vi "Dummy TVC.vi"() -> ()   [LabVIEW 2025]
uses:
  controls/TED4015 Status.ctl
  <vilib>/addons/_JKI Toolkits/State Machine/_JKI_lib_State_Machine.llb/Select State(s)_err__jki_lib_state_machine.vi
  <vilib>/addons/_JKI Toolkits/State Machine/_JKI_lib_State_Machine.llb/Periodic Trigger__ogtk__JKI-SM__jki_lib_state_machine.vi
panel:
  in  "LED_Stimulate":bool
  in  "LED_Illuminate":bool
  in  "Heater Enable":bool
  in  "PSU Enable":bool
  in  "TLUP_Temperatures":waveform(dbl)[](array[waveform])=[{"t0"=timestamp(3820413812.102944 s since 1904-01-01), "dt"=1.0, "Y"=[23.56152], "attributes"=variant("NI_ChannelName"=variant(string "TLUP_0"))}, {"t0"=timestamp(3820413812.102944 s since 1904-01-01), "dt"=1.0, "Y"=[-999.0], "attributes"=variant("NI_ChannelName"=variant(string "TLUP_1"))}, {"t0"=timestamp(3820413812.102944 s since 1904-01-01), "dt"=1.0, "Y"=[-999.0], "attributes"=variant("NI_ChannelName"=variant(string "TLUP_2"))}, {"t0"=timestamp(3820413812.102944 s since 1904-01-01), "dt"=1.0, "Y"=[-999.0], "attributes"=variant("NI_ChannelName"=variant(string "TLUP_3"))}, {"t0"=timestamp(3820413812.102944 s since 1904-01-01), "dt"=1.0, "Y"=[nan], "attributes"=variant("NI_ChannelName"=variant(string "TLUP_4"))}, {"t0"=timestamp(3820413812.102944 s since 1904-01-01), "dt"=1.0, "Y"=[nan], "attributes"=variant("NI_ChannelName"=variant(string "TLUP_5"))}, {"t0"=timestamp(3820413812.102944 s since 1904-01-01), "dt"=1.0, "Y"=[nan], "attributes"=variant("NI_ChannelName"=variant(string "TLUP_6"))}, {"t0"=timestamp(3820413812.102944 s since 1904-01-01), "dt"=1.0, "Y"=[nan], "attributes"=variant("NI_ChannelName"=variant(string "TLUP_7"))}]
  in  "TEC On":bool[](array[boolean])=[FALSE, FALSE]
  in  "DS enabled?":bool
  in  "Exit":bool
  out "TVC_StopAfterCycle":bool
  out "TVC_CyclesRemaining":i32
  in  "TVC_CycleNumber":i32
  in  "Diode Currents":waveform(dbl)[](array[waveform])
  in  "TED Status":T1[](array[typedef])
  in  "PSU_Monitor":waveform(dbl)[](array[waveform])=[{"t0"=timestamp(3820413812.1099424 s since 1904-01-01), "dt"=1.0, "Y"=[2.52], "attributes"=variant("NI_ChannelName"=variant(string "Board_Voltage_0"))}, {"t0"=timestamp(3820413812.1153584 s since 1904-01-01), "dt"=1.0, "Y"=[-0.009], "attributes"=variant("NI_ChannelName"=variant(string "Board_Voltage_0"))}, {"t0"=timestamp(3820413812.1099424 s since 1904-01-01), "dt"=1.0, "Y"=[-0.017], "attributes"=variant("NI_ChannelName"=variant(string "Board_Current_0"))}, {"t0"=timestamp(3820413812.1153584 s since 1904-01-01), "dt"=1.0, "Y"=[0.0], "attributes"=variant("NI_ChannelName"=variant(string "Board_Current_0"))}]
  in  "Heater Monitor":waveform(dbl)[](array[waveform])=[{"t0"=timestamp(3820413812.092942 s since 1904-01-01), "dt"=1.0, "Y"=[-0.005], "attributes"=variant("NI_ChannelName"=variant(string "Heater_Voltage"))}, {"t0"=timestamp(3820413812.092942 s since 1904-01-01), "dt"=1.0, "Y"=[-0.002], "attributes"=variant("NI_ChannelName"=variant(string "Heater_Current"))}]
  in  "TVC_Temperatures":waveform(dbl)[](array[waveform])=[{"t0"=timestamp(3820413812.1049423 s since 1904-01-01), "dt"=1.0, "Y"=[-80.0], "attributes"=variant("NI_ChannelName"=variant(string "3A"))}, {"t0"=timestamp(3820413812.1049423 s since 1904-01-01), "dt"=1.0, "Y"=[0.1969585335155295], "attributes"=variant("NI_ChannelName"=variant(string "3B"))}, {"t0"=timestamp(3820413812.1049423 s since 1904-01-01), "dt"=1.0, "Y"=[0.2898606356704896], "attributes"=variant("NI_ChannelName"=variant(string "3C"))}, {"t0"=timestamp(3820413812.1049423 s since 1904-01-01), "dt"=1.0, "Y"=[0.3274623555028864], "attributes"=variant("NI_ChannelName"=variant(string "3D"))}, {"t0"=timestamp(3820413812.1049423 s since 1904-01-01), "dt"=1.0, "Y"=[0.3794250746071903], "attributes"=variant("NI_ChannelName"=variant(string "4A"))}, {"t0"=timestamp(3820413812.1049423 s since 1904-01-01), "dt"=1.0, "Y"=[0.7650917242886434], "attributes"=variant("NI_ChannelName"=variant(string "4B"))}, {"t0"=timestamp(3820413812.1049423 s since 1904-01-01), "dt"=1.0, "Y"=[0.4416685188806395], "attributes"=variant("NI_ChannelName"=variant(string "4C"))}, {"t0"=timestamp(3820413812.1049423 s since 1904-01-01), "dt"=1.0, "Y"=[0.7497510727682433], "attributes"=variant("NI_ChannelName"=variant(string "4D"))}, {"t0"=timestamp(3820413812.1049423 s since 1904-01-01), "dt"=1.0, "Y"=[0.8015992709050663], "attributes"=variant("NI_ChannelName"=variant(string "Target"))}]
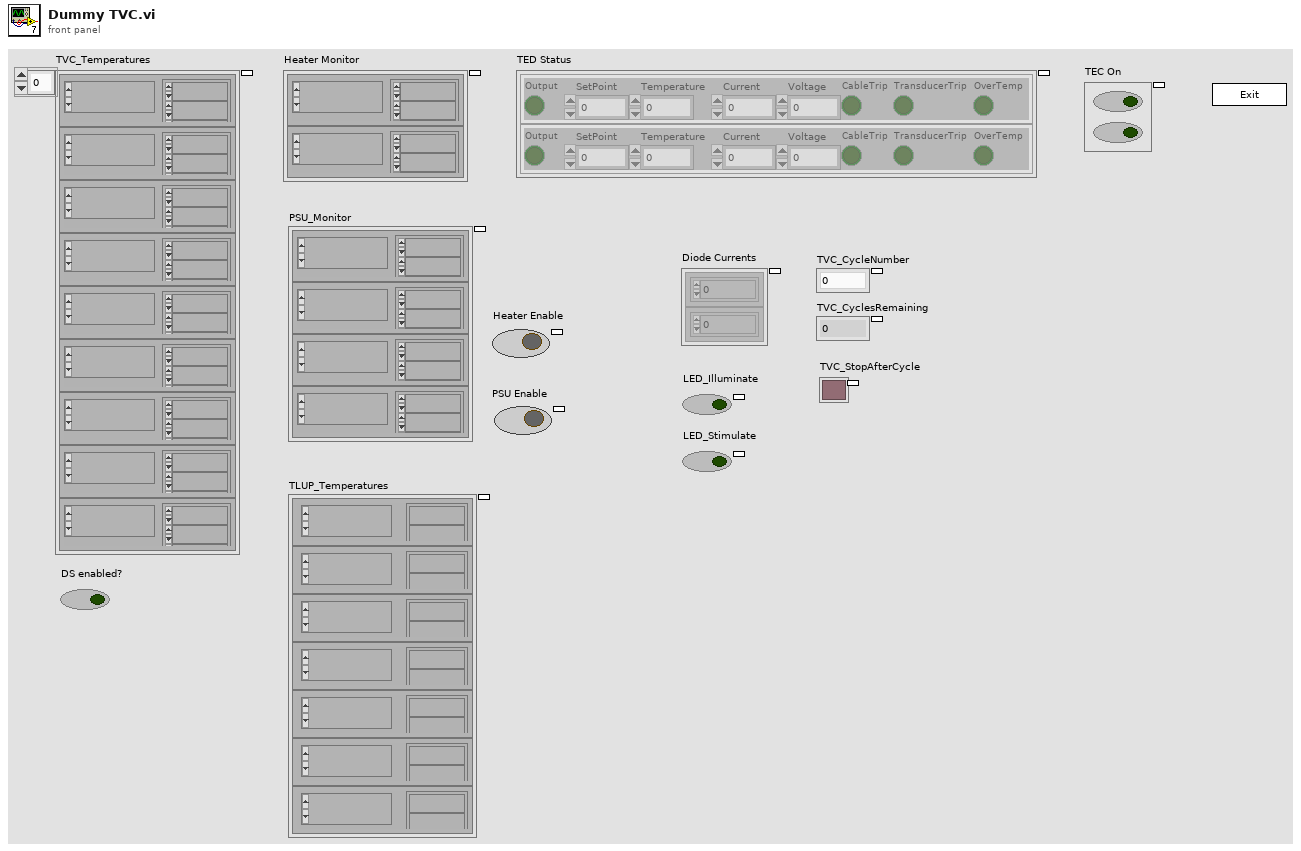
[diagram p1: front panel]
types:
  T1 = typedef "TED4015 Status.ctl" = cluster{"Output":bool, "SetPoint":dbl, "Temperature":dbl, "Current":dbl, "Voltage":dbl, "CableTrip":bool, "TransducerTrip":bool, "OverTemp":bool}
  T2 = enum32{"Invalid", "Standard", "Closed", "Hidden", "Minimized", "Maximized"}
  T3 = enum32{"invalid app kind", "Development System", "Run Time System", "Student Edition", "Embedded LabVIEW", "Evaluation", "Custom"}
  T4 = cluster{"Core":cluster{"Current VI Reference":refnum<vi>, "Close Panel on Exit?":bool}, "Your Boolean data":bool, "Your string data":string}
  T5 = cluster{"Current VI Reference":refnum<vi>, "Close Panel on Exit?":bool}
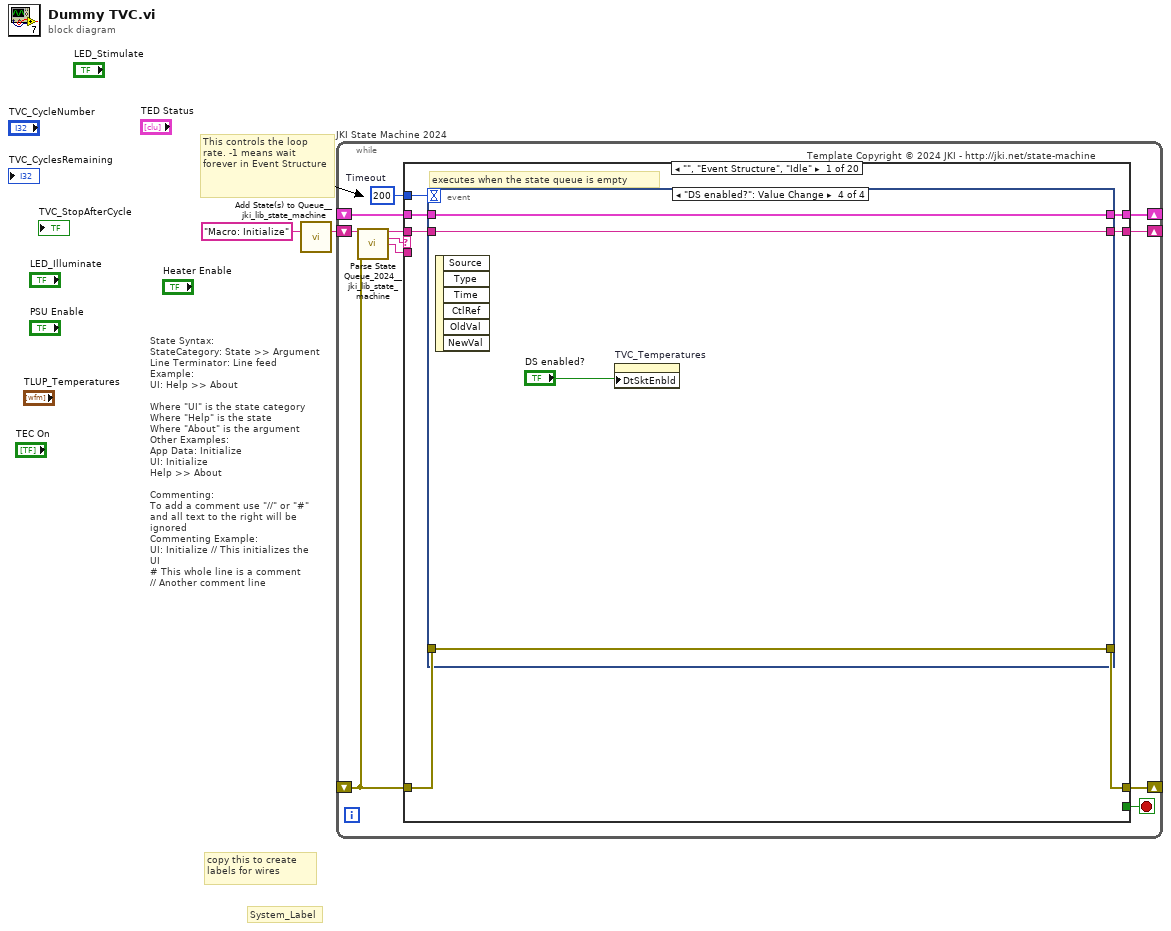
[diagram p0: block diagram]
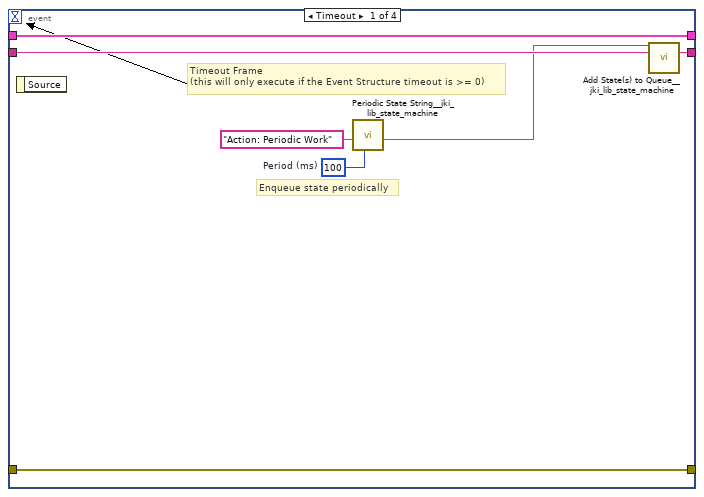
[diagram p2: hidden frame]
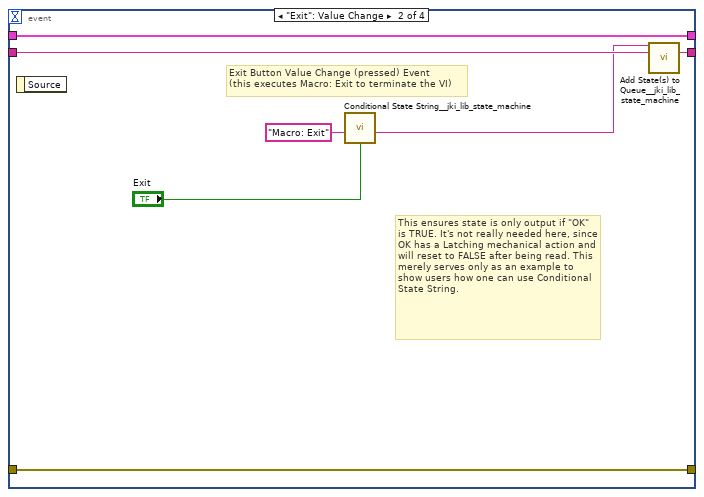
[diagram p3: hidden frame]
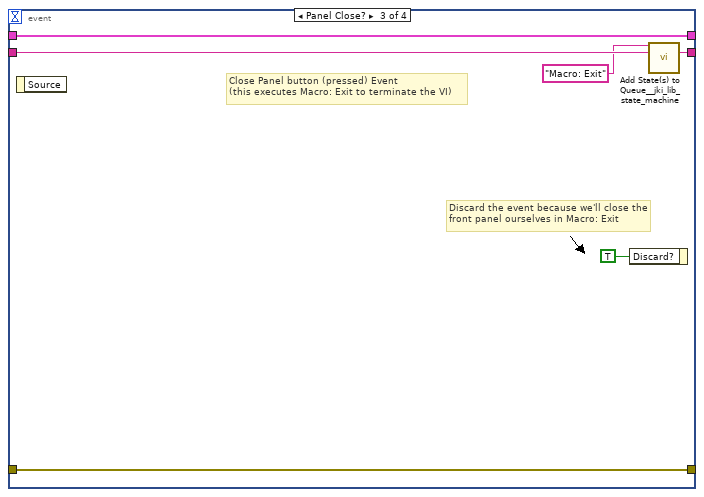
[diagram p4: hidden frame]
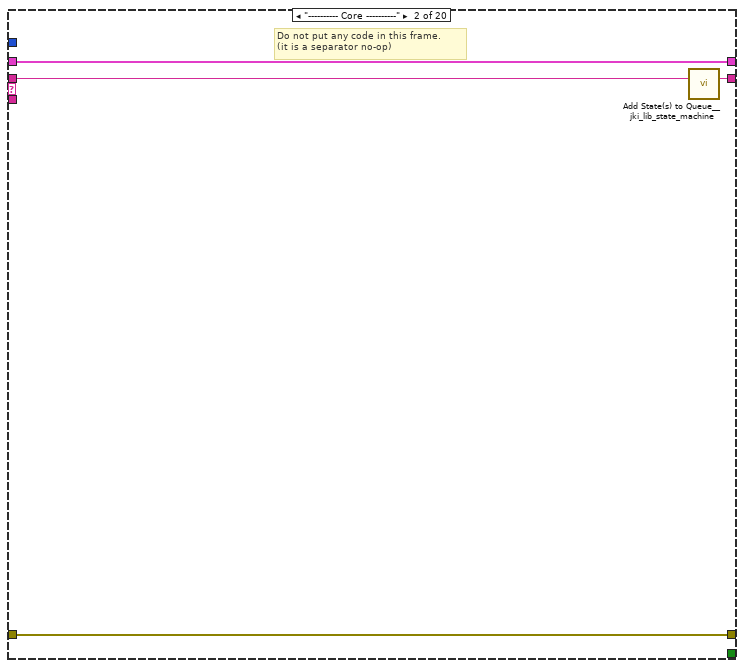
[diagram p5: hidden frame]
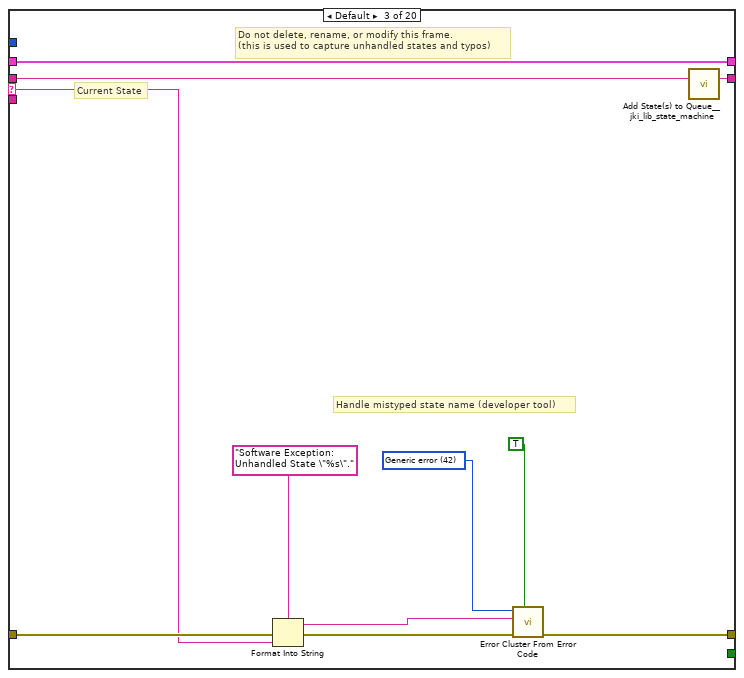
[diagram p6: hidden frame]
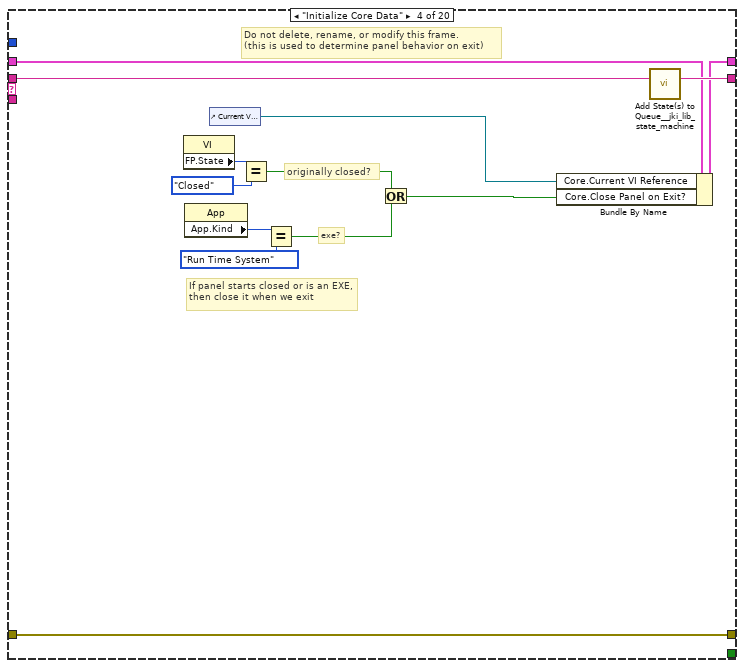
[diagram p7: hidden frame]
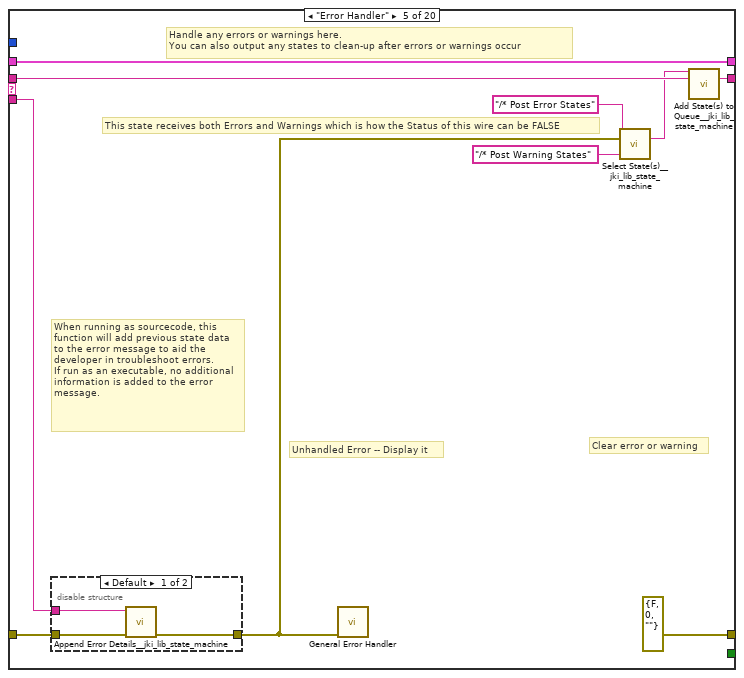
[diagram p8: hidden frame]
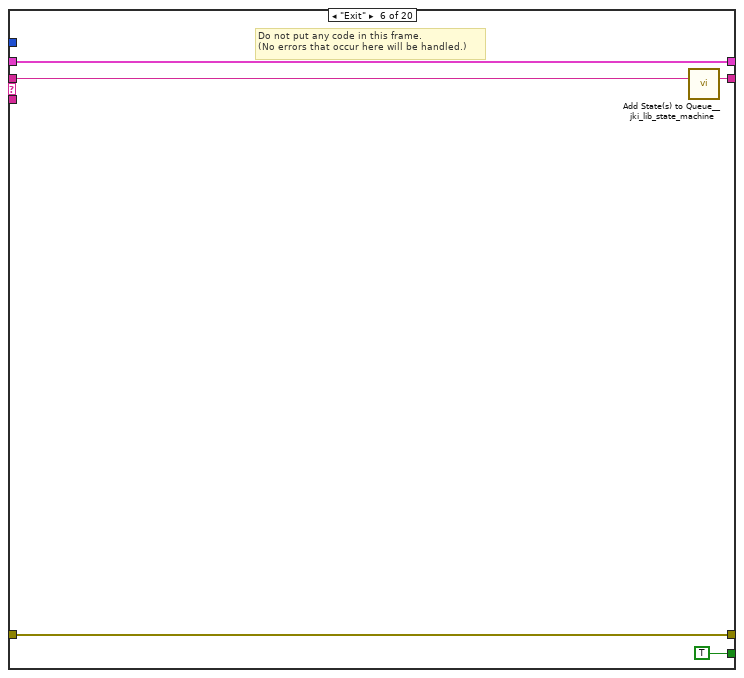
[diagram p10: hidden frame]
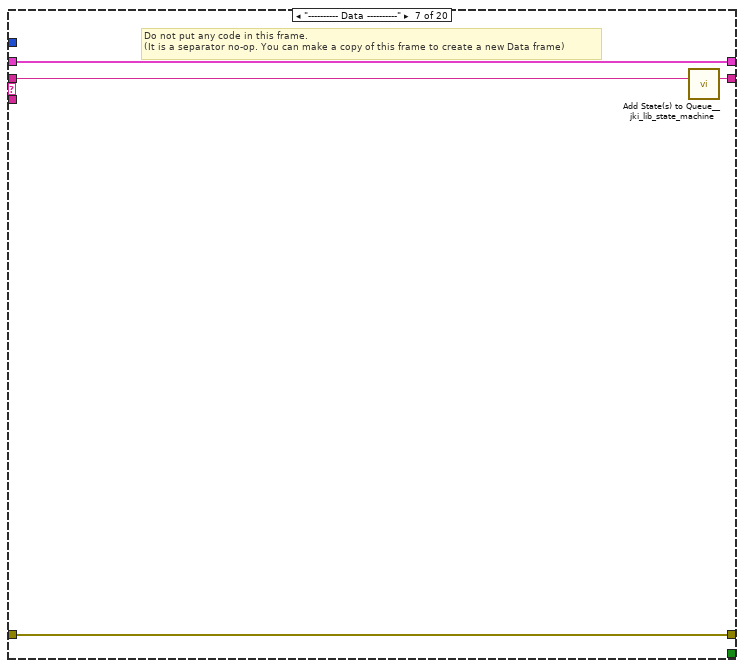
[diagram p11: hidden frame]
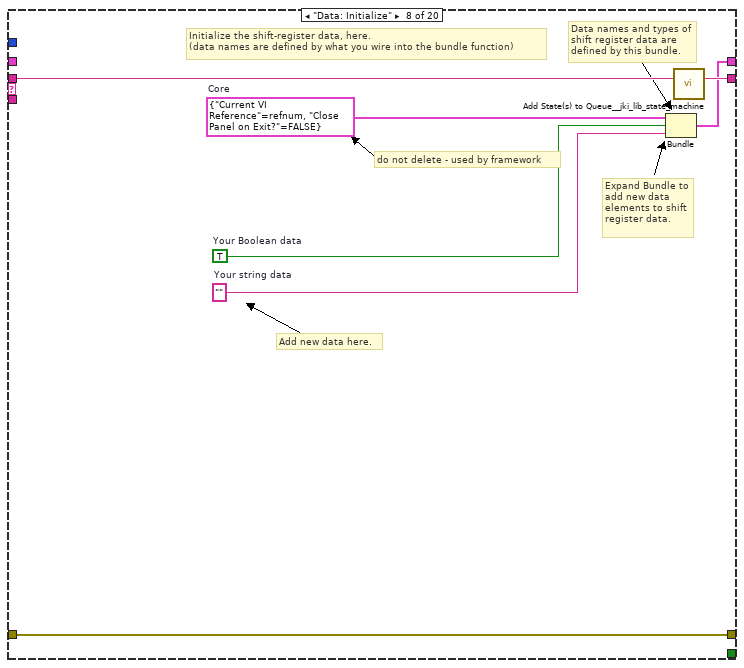
[diagram p12: hidden frame]
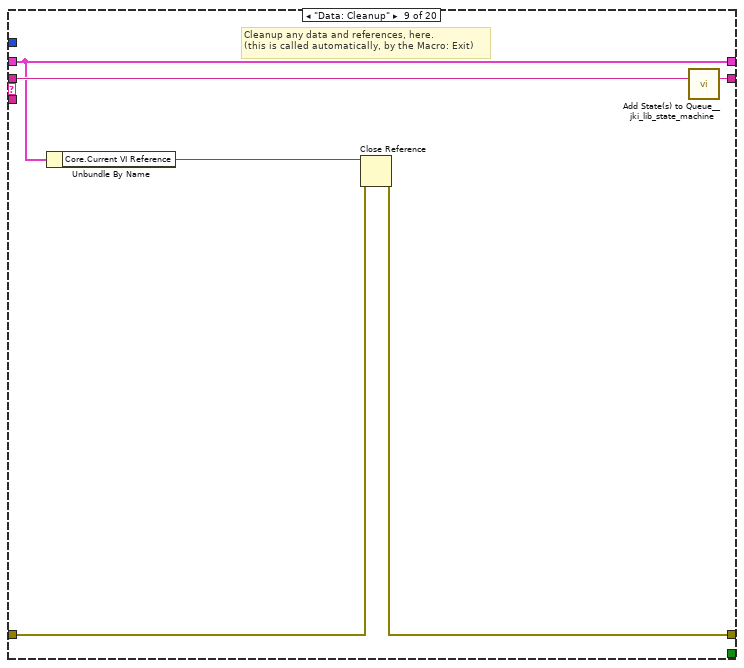
[diagram p13: hidden frame]
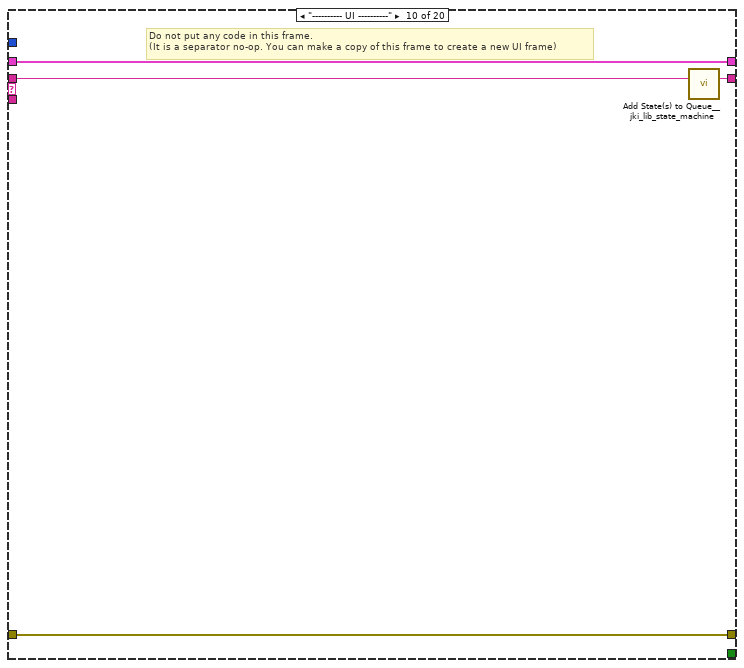
[diagram p14: hidden frame]
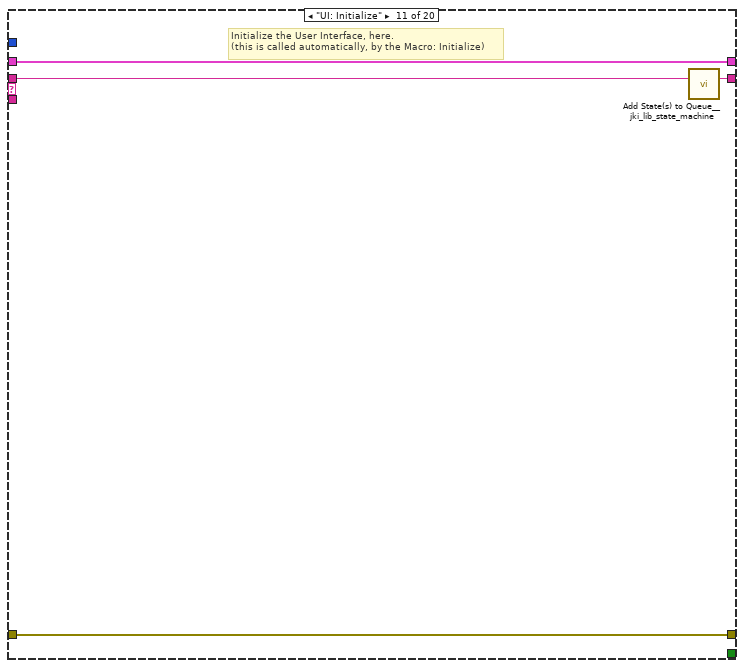
[diagram p15: hidden frame]
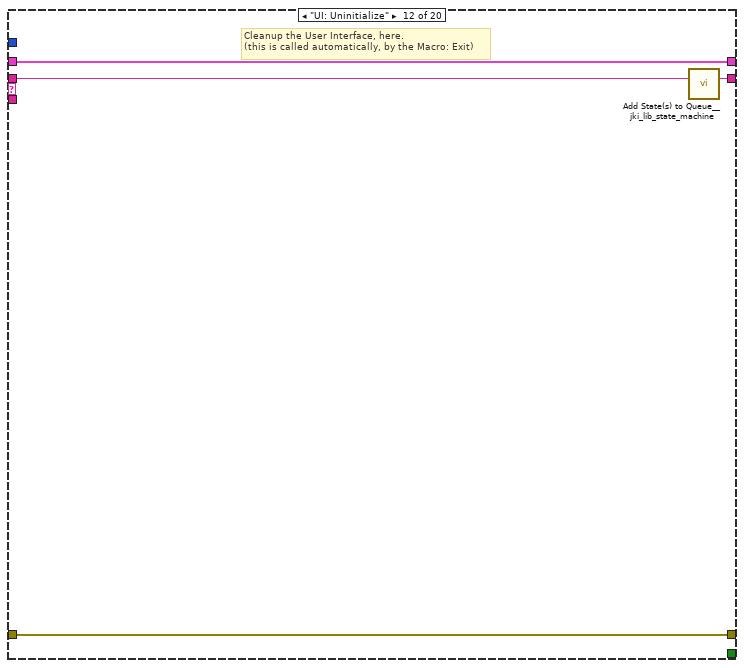
[diagram p16: hidden frame]
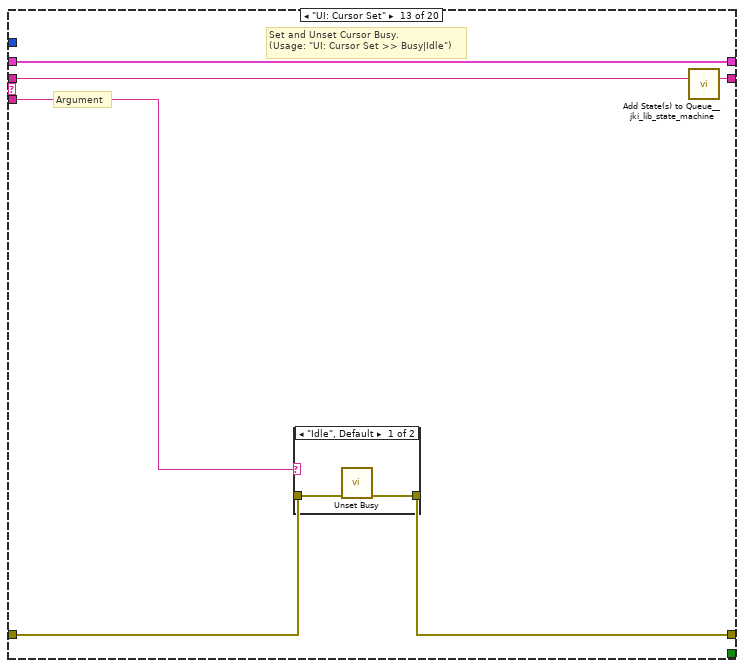
[diagram p17: hidden frame]
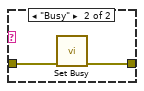
[diagram p18: hidden frame]
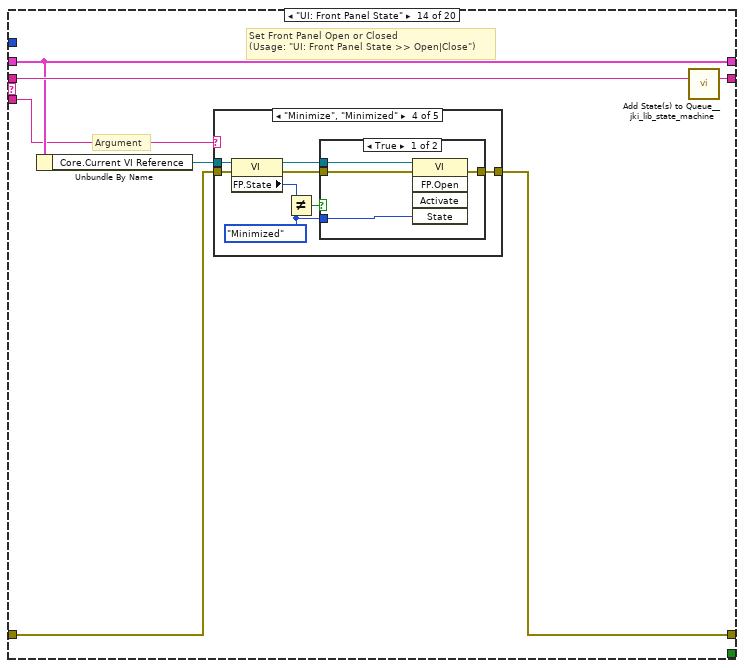
[diagram p19: hidden frame]
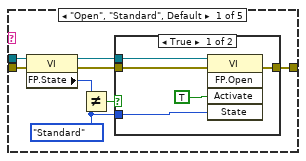
[diagram p20: hidden frame]
diagram:
  # "State Syntax:\nStateCategory: State >> Argument\nLine Terminator: Line feed\nExample:\nUI: Help >> About\n\nWhere \"UI\" is the state category\nWhere \"Help\" is the state\nWhere \"About\" is the argument\nOther Examples:\nApp Data: Initialize\nUI: Initialize\nHelp >> About\n\nCommenting:\nTo add a comment use \"//\" or \"#\" and all text to the right will be ignored\nCommenting Example:\nUI: Initialize // This initializes the UI\n# This whole line is a comment\n// Another comment line"
  # "copy this to create labels for wires"
  # "This controls the loop rate. -1 means wait forever in Event Structure"
  # "System_Label"
  n1 = call <vilib>:"Add State(s) to Queue__jki_lib_state_machine.vi"("State(s) in (\"\")"="Macro: Initialize") -> ("States Out"=w2:string)  [unwired: 14 in]
  n2 = while "JKI State Machine 2024" {
    shift-right: [w6] -> _
    shift-left: _ -> [w5]
    shift-right: [w9] -> _
    shift-left: _ -> [w3]
    shift-right: [w8] -> _
    shift-left: w2 -> [w10]
    stop <- w7 stop-if-true
    w4 = 200  # Timeout
    # "Template Copyright © 2024 JKI - http://jki.net/state-machine"
    n3 = call <vilib>:"Parse State Queue_2024__jki_lib_state_machine.vi"("State Queue"=w10, "Error In (no error)"=w3) -> ("Remaining States"=w12:string, "Current State"=w13:string, "Arguments"=w11:string)  [unwired: 11 in]
    n4 = case shown="\"\", \"Event Structure\", \"Idle\"" w13 {
      selector: w13 -> [_ _ w49 _ _ _ _ _ _ _ _ _ _ _ _ _ _ _ _ _]
      tunnel: w12 -> [w20 w48 w53 w72 w82 w91 w95 w102 w108 w112 w116 w120 w126 w137 w206 w211 w220 w224 w236 w252]
      tunnel: w11 -> [_ _ _ _ w77 _ _ _ _ _ _ _ w121 w131 _ _ _ _ _ _]
      tunnel: w5 -> [w18 w45 w51 w65 w79 w89 w92 _ w103 w109 w114 w118 w124 w133 w203 w208 w218 w221 w233 w249]
      tunnel: [w17 w46 w55 w69 errorcluster {"status"=FALSE, "code"=0, "source"=""} ("error out") w88 w93 w99 w104 w110 w113 w117 w122 w134 w204 w209 w215 w222 w234 w250] -> w9
      tunnel: w3 -> [w14 w46 w54 w69 w78 w88 w93 w99 w105 w110 w113 w117 w123 w135 w204 w209 w215 w222 w234 w250]
      tunnel: [w19 w47 w52 w71 w81 w90 w94 w101 w107 w111 w115 w119 w125 w136 w205 w210 w219 w223 w235 w251] -> w8
      tunnel: [_ _ _ _ _ TRUE _ _ _ _ _ _ _ _ _ _ _ _ _ _] -> w7
      tunnel: [w16 w45 w51 w70 w79 w89 w92 w100 w103 w109 w114 w118 w124 w133 w203 w208 w218 w221 w233 w249] -> w6
      tunnel: w4 -> [w15 _ _ _ _ _ _ _ _ _ _ _ _ _ _ _ _ _ _ _]
      frame "", "Event Structure", "Idle" {
        # "executes when the state queue is empty"
        n5 = event shown="[3] \"DS enabled?\": Value Change" {
          selector: _ -> [_ _ _ _]
          dyn-events: _ -> [_ _ _ _]
          timeout: w15 -> [_ _ _ _]
          tunnel: w20 -> [w27 w34 w40 w43]
          tunnel: [w26 w33 w39 w43] -> w19
          tunnel: w18 -> [w24 w31 w37 w44]
          tunnel: [w25 w32 w38 w42] -> w17
          tunnel: w14 -> [w25 w32 w38 w42]
          tunnel: [w24 w31 w37 w44] -> w16
          event Timeout {
            w21 = u32 100  # Period (ms)
            # "Enqueue state periodically"
            # "Timeout Frame\n(this will only execute if the Event Structure timeout is >= 0)"
            n6 = event-data() -> ()  [unwired: 1 in, 1 out]
            n7 = call <vilib>:"Periodic State String__jki_lib_state_machine.vi"("Period (ms)"=w21, "State"="Action: Periodic Work") -> ("State Out"=w23:string)  [unwired: 9 in]
            n8 = call <vilib>:"Add State(s) to Queue__jki_lib_state_machine.vi"("State(s) in Front (\"\")"=w23, "State(s) in (\"\")"=w27) -> ("States Out"=w26:string)  [unwired: 13 in]
          }
          event "Exit": Value Change {
            # "This ensures state is only output if \"OK\" is TRUE. It's not really needed here, since OK has a Latching mechanical action and will reset to FALSE after being read. This merely serves only as an example to show users how one can use Conditional State String."
            # "Exit Button Value Change (pressed) Event\n(this executes Macro: Exit to terminate the VI)"
            n9 = event-data() -> ()  [unwired: 1 in, 1 out]
            n10 = call <vilib>:"Conditional State String__jki_lib_state_machine.vi"("Do State(s)?"="Exit", "State"="Macro: Exit") -> ("State Out"=w28:string)  [unwired: 7 in]
            n11 = call <vilib>:"Add State(s) to Queue__jki_lib_state_machine.vi"("State(s) in Front (\"\")"=w28, "State(s) in (\"\")"=w34) -> ("States Out"=w33:string)  [unwired: 13 in]
          }
          event Panel Close? {
            # "Discard the event because we'll close the front panel ourselves in Macro: Exit"
            # "Close Panel button (pressed) Event\n(this executes Macro: Exit to terminate the VI)"
            n12 = event-data() -> ()  [unwired: 1 in, 1 out]
            n13 = event-data("Discard?"=TRUE) -> ()  [unwired: 1 in, 1 out]
            n14 = call <vilib>:"Add State(s) to Queue__jki_lib_state_machine.vi"("State(s) in Front (\"\")"="Macro: Exit", "State(s) in (\"\")"=w40) -> ("States Out"=w39:string)  [unwired: 13 in]
          }
          event "DS enabled?": Value Change {
            n15 = event-data() -> ()  [unwired: 1 in, 6 out]
            n16 = property on="TVC_Temperatures" class="Arr (strict)"("DtSktEnbld"="DS enabled?") -> ()  [unwired: 2 in, 2 out]
          }
        }
      }
      frame "---------- Core ----------" {
        # "Do not put any code in this frame.\n(it is a separator no-op)"
        n17 = call <vilib>:"Add State(s) to Queue__jki_lib_state_machine.vi"("State(s) in (\"\")"=w48) -> ("States Out"=w47:string)  [unwired: 14 in]
      }
      frame Default {
        w58 = 42 items=["No error", "Argument error", "Memory is full", "Out of zone", "End of file", "File already open", "Generic file I/O error", "File not found", "File permission error", "Disk is full", "Duplicate path", "Too many files open", "System feature not enabled", "Resource file not found", "Cannot add resource", "Resource not found", "Image not found", "Image memory error", "Pen does not exist", "Config type invalid", "Config token not found", "Config parse error", "Config memory error", "Bad external code format", "Bad external code offset", "External code not present", "Null window", "Destroy window error", "Null menu", "Print aborted", "Bad print record", "Print driver error", "Windows error during printing", "Memory error during printing", "Print dialog error", "Generic print error", "Invalid device refnum", "Device not found", "Device parameter error", "Device unit error", "Cannot open device", "Device call aborted", "Generic error", "Cancelled by user", "Object ID too low", "Object ID too high", "Object not in heap", "Unknown heap", "Unknown object (invalid DefProc)", "Unknown object (DefProc not in table)", "Message out of range", "Invalid (null) method", "Unknown message", "Manager call not supported", "Bad address", "Network operation in progress", "Network operation timed out", "Connection is busy", "Network attribute not supported", "Network error", "Address in use", "System out of memory", "Connection aborted", "Connection refused", "Not connected", "Already connected", "Connection closed", "Initialization error (interapplication manager)", "Bad occurrence", "Wait on unbound occurrence handler", "Occurrence queue overflow", "Datalog type conflict", "Unused", "Unrecognized type (interapplication manager)", "Memory corrupt", "Failed to make temporary DLL", "Old CIN version", "Drag socket not found", "Failed to load drop-object", "Failed to register OLE object", "Failed to release OLE object", "Format specifier type mismatch", "Unknown format specifier", "Too few format specifiers", "Too many format specifiers", "Scan failed", "Newer CIN version", "Error converting to variant", "Runtime menu error", "Password tampered", "Variant attribute not found", "Incompatible variant data type", "Event data is not available", "Event Store is not present", "Occurrence is not found", "Event Queue is not created", "Event info is not available", "Refnum passed is NULL", "Error retrieving Class GUID", "Error retrieving CoClass GUID", "Error retrieving TypeLib GUID.", "Bad built application magic bytes.", "Specific driver is different from the specific driver associated with the Logical Name.", "There is no session opened to the class driver.", "Max Error", "MAX - Error with config objects", "MAX - Error loading configuration", "MAX - Group not supported"]
        # "Current State"
        # "Do not delete, rename, or modify this frame.\n(this is used to capture unhandled states and typos)"
        # "Handle mistyped state name (developer tool)"
        n18 = Format Into String(format string="Software Exception: Unhandled State \"%s\"." ("message"), error in=w54, w49) -> (resulting string=w57:string, error out=w56:errorcluster)  [unwired: 1 in]
        n19 = call <vilib>:"Error Cluster From Error Code.vi"("show call chain? (False)"=TRUE, "error in (no error)"=w56, "error message (\"\")"=w57, "error code (0)"=w58) -> ("error out"=w55:errorcluster)  [unwired: 5 in]
        n20 = call <vilib>:"Add State(s) to Queue__jki_lib_state_machine.vi"("State(s) in (\"\")"=w53) -> ("States Out"=w52:string)  [unwired: 14 in]
      }
      frame "Initialize Core Data" {
        # "Do not delete, rename, or modify this frame.\n(this is used to determine panel behavior on exit)"
        # "originally closed?"
        # "exe?"
        # "If panel starts closed or is an EXE, then close it when we exit"
        n21 = property class="VI"() -> ("FP.State"=w62:T2)  [unwired: 2 in, 2 out]
        n22 = property class="App"() -> ("App.Kind"=w68:T3)  [unwired: 2 in, 2 out]
        n23 = control-ref of="Current VI Reference"() -> (w63:refnum<vi>)
        n24 = Equal?(x=w62, y=T2."Closed" ("Front Panel Window:State")) -> (x = y?=w60:bool)
        n25 = Equal?(x=w68, y=T3."Run Time System" ("Application:Kind")) -> (x = y?=w66:bool)
        n26 = Or(x=w60, y=w66) -> (x .or. y?=w64:bool)
        n27 = Bundle By Name(cluster=w65, "Core.Current VI Reference"=w63, "Core.Close Panel on Exit?"=w64) -> (w70:T4)
        n28 = call <vilib>:"Add State(s) to Queue__jki_lib_state_machine.vi"("State(s) in (\"\")"=w72) -> ("States Out"=w71:string)  [unwired: 14 in]
      }
      frame "Error Handler" {
        # "When running as sourcecode, this function will add previous state data to the error message to aid the developer in troubleshoot errors.\nIf run as an executable, no additional information is added to the error message."
        # "This state receives both Errors and Warnings which is how the Status of this wire can be FALSE"
        # "Unhandled Error -- Display it"
        # "Handle any errors or warnings here.\nYou can also output any states to clean-up after errors or warnings occur"
        # "Clear error or warning"
        n29 = disable-structure shown="Default" {
          disable-tunnel: w78 -> [w85 w86]
          disable-tunnel: w77 -> [w84 _]
          disable-tunnel: [w83 w86] -> w76
          frame condition #0 (active) {
            n30 = call <vilib>:"Append Error Details__jki_lib_state_machine.vi"("error in (no error)"=w85, "Previous State and Argument(s)"=w84) -> ("error out"=w83:errorcluster)  [unwired: 9 in]
          }
          frame condition #1 {
          }
        }
        n31 = call <vilib>:"General Error Handler.vi"("error in (no error)"=w76) -> ()  [unwired: 10 in, 5 out]
        n32 = call-poly <vilib>:"Select State(s)__jki_lib_state_machine.vi"("State(s) if True (\"\")"="/* Post Error States", "Select"=w76, "State(s) if False (\"\")"="/* Post Warning States") -> ("States Out"=w74:string)  [unwired: 12 in]
        n33 = call <vilib>:"Add State(s) to Queue__jki_lib_state_machine.vi"("State(s) in Front (\"\")"=w74, "State(s) in (\"\")"=w82) -> ("States Out"=w81:string)  [unwired: 13 in]
      }
      frame "Exit" {
        # "Do not put any code in this frame.\n(No errors that occur here will be handled.)"
        n34 = call <vilib>:"Add State(s) to Queue__jki_lib_state_machine.vi"("State(s) in (\"\")"=w91) -> ("States Out"=w90:string)  [unwired: 14 in]
      }
      frame "---------- Data ----------" {
        # "Do not put any code in this frame.\n(It is a separator no-op. You can make a copy of this frame to create a new Data frame)"
        n35 = call <vilib>:"Add State(s) to Queue__jki_lib_state_machine.vi"("State(s) in (\"\")"=w95) -> ("States Out"=w94:string)  [unwired: 14 in]
      }
      frame "Data: Initialize" {
        w96 = T5 {"Current VI Reference"=refnum, "Close Panel on Exit?"=FALSE}  # Core
        w98 = TRUE  # Your Boolean data
        w97 = ""  # Your string data
        # "do not delete - used by framework"
        # "Expand Bundle to add new data elements to shift register data."
        # "Add new data here."
        # "Data names and types of shift register data are defined by this bundle."
        # "Initialize the shift-register data, here.\n(data names are defined by what you wire into the bundle function)"
        n36 = Bundle("Core"=w96, "Your Boolean data"=w98, "Your string data"=w97) -> (w100:T4)  [unwired: 1 in]
        n37 = call <vilib>:"Add State(s) to Queue__jki_lib_state_machine.vi"("State(s) in (\"\")"=w102) -> ("States Out"=w101:string)  [unwired: 14 in]
      }
      frame "Data: Cleanup" {
        # "Cleanup any data and references, here.\n(this is called automatically, by the Macro: Exit)"
        n38 = Unbundle By Name(w103) -> ("Core.Current VI Reference"=w106:refnum<vi>)
        n39 = Close Reference(reference=w106, error in (no error)=w105) -> (error out=w104:errorcluster)
        n40 = call <vilib>:"Add State(s) to Queue__jki_lib_state_machine.vi"("State(s) in (\"\")"=w108) -> ("States Out"=w107:string)  [unwired: 14 in]
      }
      frame "---------- UI ----------" {
        # "Do not put any code in this frame.\n(It is a separator no-op. You can make a copy of this frame to create a new UI frame)"
        n41 = call <vilib>:"Add State(s) to Queue__jki_lib_state_machine.vi"("State(s) in (\"\")"=w112) -> ("States Out"=w111:string)  [unwired: 14 in]
      }
      frame "UI: Initialize" {
        # "Initialize the User Interface, here.\n(this is called automatically, by the Macro: Initialize)"
        n42 = call <vilib>:"Add State(s) to Queue__jki_lib_state_machine.vi"("State(s) in (\"\")"=w116) -> ("States Out"=w115:string)  [unwired: 14 in]
      }
      frame "UI: Uninitialize" {
        # "Cleanup the User Interface, here.\n(this is called automatically, by the Macro: Exit)"
        n43 = call <vilib>:"Add State(s) to Queue__jki_lib_state_machine.vi"("State(s) in (\"\")"=w120) -> ("States Out"=w119:string)  [unwired: 14 in]
      }
      frame "UI: Cursor Set" {
        # "Argument"
        # "Set and Unset Cursor Busy.\n(Usage: \"UI: Cursor Set >> Busy|Idle\")"
        n44 = case shown="\"Idle\", Default" w121 {
          tunnel: w123 -> [w128 w130]
          tunnel: [w127 w129] -> w122
          frame "Idle", Default {
            n45 = call <vilib>:"Unset Busy.vi"("error in (no error)"=w128) -> ("error out"=w127:errorcluster)  [unwired: 10 in]
          }
          frame "Busy" {
            n46 = call <vilib>:"Set Busy.vi"("error in (no error)"=w130) -> ("error out"=w129:errorcluster)  [unwired: 9 in, 1 out]
          }
        }
        n47 = call <vilib>:"Add State(s) to Queue__jki_lib_state_machine.vi"("State(s) in (\"\")"=w126) -> ("States Out"=w125:string)  [unwired: 14 in]
      }
      frame "UI: Front Panel State" {
        # "Argument"
        # "Set Front Panel Open or Closed\n(Usage: \"UI: Front Panel State >> Open|Close\")"
        n48 = Unbundle By Name(w133) -> ("Core.Current VI Reference"=w132:refnum<vi>)
        n49 = case shown="\"Minimize\", \"Minimized\"" w131 {
          tunnel: w135 -> [w143 w158 w169 w182 w195]
          tunnel: [w145 w159 w171 w184 w197] -> w134
          tunnel: w132 -> [w144 w156 w170 w183 w196]
          frame "Open", "Standard", Default {
            w138 = T2."Standard" ("State")
            n50 = property class="VI"(reference=w144, error in=w143) -> (reference out=w141:refnum<vi>, error out=w142:errorcluster, "FP.State"=w140:T2)
            n51 = Not Equal?(x=w140, y=w138) -> (x != y?=w139:bool)
            n52 = case shown="True" w139 {
              tunnel: [w149 w151] -> w145
              tunnel: w142 -> [w148 w151]
              tunnel: w141 -> [w147 _]
              tunnel: w138 -> [w146 _]
              frame True {
                n53 = invoke class="VI" method="FP.Open"(reference=w147, error in=w148, "Activate"=TRUE, "State"=w146) -> (error out=w149:errorcluster)  [unwired: 1 in, 4 out]
              }
              frame False {
              }
            }
          }
          frame "Close", "Closed" {
            n54 = property class="VI"(reference=w156, error in=w158) -> (reference out=w155:refnum<vi>, error out=w157:errorcluster, "FP.State"=w153:T2)
            n55 = Not Equal?(x=w153, y=T2."Closed" ("Front Panel Window:State")) -> (x != y?=w152:bool)
            n56 = case shown="True" w152 {
              tunnel: [w160 w163] -> w159
              tunnel: w157 -> [w160 w162]
              tunnel: w155 -> [_ w161]
              frame False {
              }
              frame True {
                n57 = invoke class="VI" method="FP.Close"(reference=w161, error in=w162) -> (error out=w163:errorcluster)  [unwired: 1 in, 2 out]
              }
            }
          }
          frame "Hidden", "Hide" {
            w164 = T2."Hidden" ("State")
            n58 = property class="VI"(reference=w170, error in=w169) -> (reference out=w167:refnum<vi>, error out=w168:errorcluster, "FP.State"=w166:T2)
            n59 = Not Equal?(x=w166, y=w164) -> (x != y?=w165:bool)
            n60 = case shown="True" w165 {
              tunnel: [w175 w176] -> w171
              tunnel: w168 -> [w174 w176]
              tunnel: w167 -> [w173 _]
              tunnel: w164 -> [w172 _]
              frame True {
                n61 = invoke class="VI" method="FP.Open"(reference=w173, error in=w174, "State"=w172) -> (error out=w175:errorcluster)  [unwired: 2 in, 4 out]
              }
              frame False {
              }
            }
          }
          frame "Minimize", "Minimized" {
            w177 = T2."Minimized" ("State")
            n62 = property class="VI"(reference=w183, error in=w182) -> (reference out=w180:refnum<vi>, error out=w181:errorcluster, "FP.State"=w179:T2)
            n63 = Not Equal?(x=w179, y=w177) -> (x != y?=w178:bool)
            n64 = case shown="True" w178 {
              tunnel: [w188 w189] -> w184
              tunnel: w181 -> [w187 w189]
              tunnel: w180 -> [w186 _]
              tunnel: w177 -> [w185 _]
              frame True {
                n65 = invoke class="VI" method="FP.Open"(reference=w186, error in=w187, "State"=w185) -> (error out=w188:errorcluster)  [unwired: 2 in, 4 out]
              }
              frame False {
              }
            }
          }
          frame "Maximize", "Maximized" {
            w190 = T2."Maximized" ("State")
            n66 = property class="VI"(reference=w196, error in=w195) -> (reference out=w193:refnum<vi>, error out=w194:errorcluster, "FP.State"=w192:T2)
            n67 = Not Equal?(x=w192, y=w190) -> (x != y?=w191:bool)
            n68 = case shown="True" w191 {
              tunnel: [w201 w202] -> w197
              tunnel: w194 -> [w200 w202]
              tunnel: w193 -> [w199 _]
              tunnel: w190 -> [w198 _]
              frame True {
                n69 = invoke class="VI" method="FP.Open"(reference=w199, error in=w200, "State"=w198) -> (error out=w201:errorcluster)  [unwired: 2 in, 4 out]
              }
              frame False {
              }
            }
          }
        }
        n70 = call <vilib>:"Add State(s) to Queue__jki_lib_state_machine.vi"("State(s) in (\"\")"=w137) -> ("States Out"=w136:string)  [unwired: 14 in]
      }
      frame "---------- Macro ----------" {
        # "Do not put any code in this frame.\n(It is a separator no-op. You can make a copy of this frame to create a new Macro frame)"
        n71 = call <vilib>:"Add State(s) to Queue__jki_lib_state_machine.vi"("State(s) in (\"\")"=w206) -> ("States Out"=w205:string)  [unwired: 14 in]
      }
      frame "Macro: Initialize" {
        w207 = "Data: Initialize\nInitialize Core Data\nUI: Initialize\nUI: Front Panel State >> Open"  # Data: Initialize Initialize Core Data UI: Initialize UI: Front Panel State >> Open
        # "Initialization Macro\n(This is called once, when the VI starts)"
        n72 = call <vilib>:"Add State(s) to Queue__jki_lib_state_machine.vi"("State(s) in Front (\"\")"=w207, "State(s) in (\"\")"=w211) -> ("States Out"=w210:string)  [unwired: 13 in]
      }
      frame "Macro: Exit" {
        # "Exit Macro\n(This is called once, when the VI exits)"
        n73 = Unbundle By Name(w218) -> ("Core.Close Panel on Exit?"=w213:bool)
        n74 = call <vilib>:"Conditional State String__jki_lib_state_machine.vi"("Do State(s)?"=w213, "State"="UI: Front Panel State >> Close") -> ("State Out"=w212:string)  [unwired: 7 in]
        n75 = call <vilib>:"Add State(s) to Queue__jki_lib_state_machine.vi"("State(s) in (\"\")"=w212, "State(s) at Back (\"\")"="UI: Uninitialize\nData: Cleanup\nExit") -> ("States Out"=w216:string)  [unwired: 13 in]
        n76 = call <vilib>:"Add State(s) to Queue__jki_lib_state_machine.vi"("State(s) in Front (\"\")"=w216, "State(s) in (\"\")"=w220) -> ("States Out"=w219:string)  [unwired: 13 in]
      }
      frame "---------- Action ----------" {
        # "Template Separator\n(You can make a copy of, or modify, this frame)"
        n77 = call <vilib>:"Add State(s) to Queue__jki_lib_state_machine.vi"("State(s) in (\"\")"=w224) -> ("States Out"=w223:string)  [unwired: 14 in]
      }
      frame "Action: Periodic Work" {
        n78 = for {
          tunnel: "PSU_Monitor" -> [w244] mode=indexing
          tunnel: [w243] -> w228 mode=indexing
          n79 = in-place {
            n80 = in-place-cluster #1(w244) -> ()  [unwired: 1 out]
            n81 = Get Date/Time In Seconds() -> (seconds since 1Jan1904=w245:timestamp)
            n82 = in-place-cluster #1("t0"=w245) -> (w243:waveform(dbl))
          }
        }
        n83 = for {
          tunnel: "TVC_Temperatures" -> [w247] mode=indexing
          tunnel: [w246] -> w226 mode=indexing
          n84 = in-place {
            n85 = in-place-cluster #2(w247) -> ()  [unwired: 1 out]
            n86 = Get Date/Time In Seconds() -> (seconds since 1Jan1904=w248:timestamp)
            n87 = in-place-cluster #2("t0"=w248) -> (w246:waveform(dbl))
          }
        }
        n88 = for {
          tunnel: "Heater Monitor" -> [w241] mode=indexing
          tunnel: [w240] -> w230 mode=indexing
          n89 = in-place {
            n90 = in-place-cluster #3(w241) -> ()  [unwired: 1 out]
            n91 = Get Date/Time In Seconds() -> (seconds since 1Jan1904=w242:timestamp)
            n92 = in-place-cluster #3("t0"=w242) -> (w240:waveform(dbl))
          }
        }
        n93 = for {
          tunnel: "Diode Currents" -> [w238] mode=indexing
          tunnel: [w237] -> w232 mode=indexing
          n94 = in-place {
            n95 = in-place-cluster #4(w238) -> ()  [unwired: 1 out]
            n96 = Get Date/Time In Seconds() -> (seconds since 1Jan1904=w239:timestamp)
            n97 = in-place-cluster #4("t0"=w239) -> (w237:waveform(dbl))
          }
        }
        n98 = property on="Heater Monitor" class="Arr (strict)"("Value"=w230) -> ()  [unwired: 2 in, 2 out]
        n99 = local write "Diode Currents"(w232) -> ()
        n100 = property on="PSU_Monitor" class="Arr (strict)"("Value"=w228) -> ()  [unwired: 2 in, 2 out]
        n101 = property on="TVC_Temperatures" class="Arr (strict)"("Value"=w226) -> ()  [unwired: 2 in, 2 out]
        n102 = call <vilib>:"Add State(s) to Queue__jki_lib_state_machine.vi"("State(s) in (\"\")"=w236) -> ("States Out"=w235:string)  [unwired: 14 in]
      }
      frame "New Category: 2" {
        # "Your code here.\n(You can make a copy of, or modify, this frame)"
        n103 = call <vilib>:"Add State(s) to Queue__jki_lib_state_machine.vi"("State(s) in (\"\")"=w252) -> ("States Out"=w251:string)  [unwired: 14 in]
      }
    }
  }
